vi "CupFinderV6.vi"() -> ()   [LabVIEW 2017]
panel:
  out "Y-Out":dbl
  out "X-Out":dbl
  out "CupPosition":T1(plugin-control)
  in  "File Path":path
  out "ImgToCrop":T1(plugin-control)
  out "Src Img":T1(plugin-control)
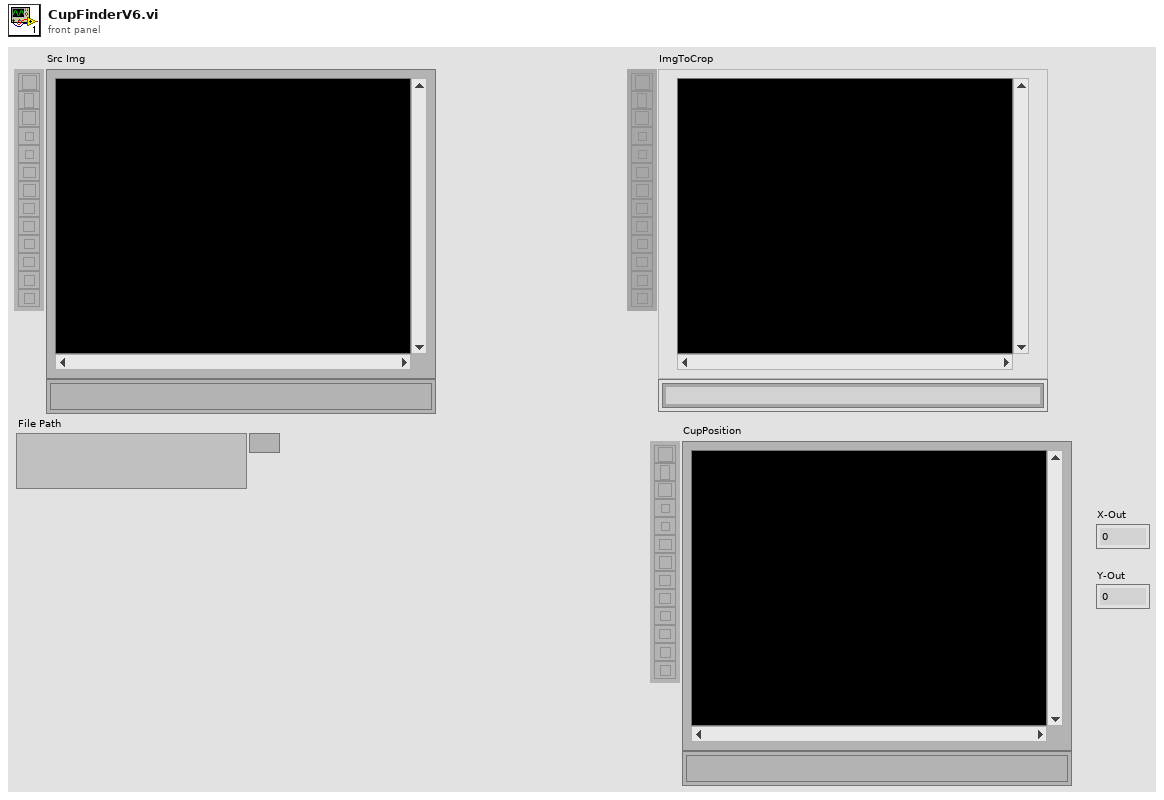
[diagram p1: front panel]
types:
  T1 = typedef "IMAQ Image.ctl" = refnum<image>
  T2 = typedef "Image Type" = u32
  T3 = cluster{"Position":cluster{"x":sgl, "y":sgl}, "Angle":sgl, "Scale":sgl, "Score":sgl, "Bounding Box":cluster{"x":sgl, "y":sgl}[]}[]
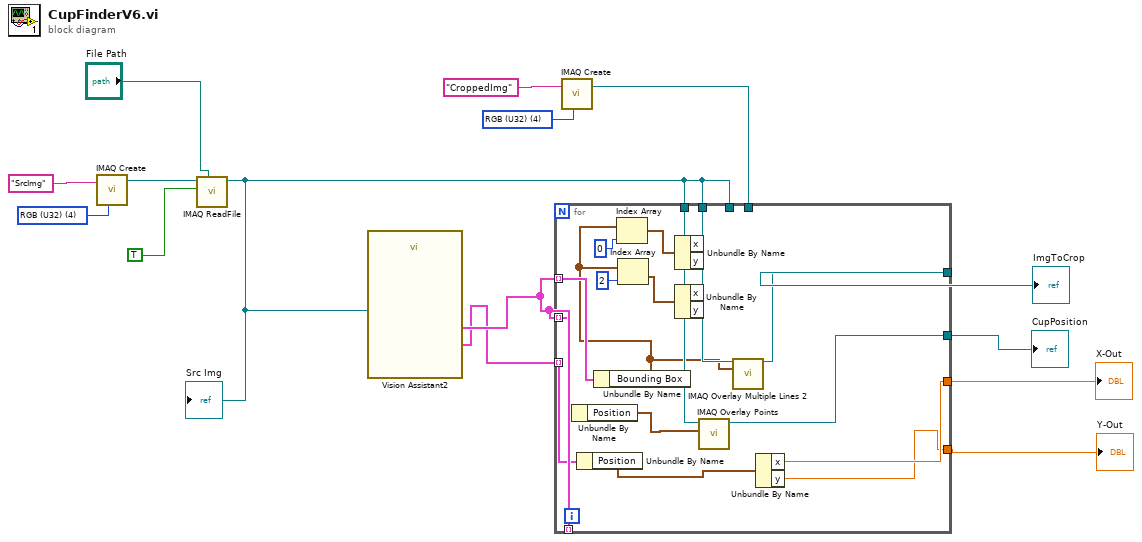
[diagram p0: block diagram]
diagram:
  w3 = T2 4 items=["Grayscale (U8)", "Grayscale (I16)", "Grayscale (SGL)", "Complex (CSG)", "RGB (U32)", "HSL (U32)", "RGB (U64)", "Grayscale (U16)"] ("Image Type")
  w14 = T2 4 items=["Grayscale (U8)", "Grayscale (I16)", "Grayscale (SGL)", "Complex (CSG)", "RGB (U32)", "HSL (U32)", "RGB (U64)", "Grayscale (U16)"] ("Image Type")
  n1 = call "IMAQ Create"("Image Name"="SrcImg", "Image Type"=w14) -> ("New Image"=w12:T1)  [unwired: 3 in, 1 out]
  n2 = call "IMAQ ReadFile"("File Path"="File Path", "Load Color Palette? (No)"=TRUE, "Image"=w12) -> ("Image Out"=w1:T1)  [unwired: 4 in, 4 out]
  "Src Img" <- w1
  n3 = call "Vision Assistant2"("Image In"=w1) -> ("Calibrated Matches (Pattern Matching 5)"=w5:T3, "Matches (Pattern Matching 5)"=w6:T3)  [unwired: 23 in, 2 out]
  n4 = call "IMAQ Create"("Image Name"="CroppedImg", "Image Type"=w3) -> ("New Image"=w2:T1)  [unwired: 3 in, 1 out]
  n5 = for {
    tunnel: [w22] -> w10
    tunnel: [w31] -> w9
    tunnel: [w29] -> w8
    tunnel: [w28] -> w7
    tunnel: w6 -> [_] mode=indexing
    tunnel: w1 -> [w27]
    tunnel: w1 -> [w26]
    tunnel: w6 -> [w24] mode=indexing
    tunnel: w6 -> [w21] mode=indexing
    tunnel: w5 -> [w23] mode=indexing
    tunnel: w2 -> [_]
    tunnel: w1 -> [_]
    n6 = Unbundle By Name(w24) -> ("Position"=w25:cluster{"x":sgl, "y":sgl})
    n7 = Unbundle By Name(w23) -> ("Position"=w30:cluster{"x":sgl, "y":sgl})
    n8 = Unbundle By Name(w21) -> ("Bounding Box"=w18:cluster{"x":sgl, "y":sgl}[])
    n9 = Index Array(array=w18, index=0) -> (element=w19:cluster{"x":sgl, "y":sgl})
    n10 = Index Array(array=w18, index=2) -> (element=w16:cluster{"x":sgl, "y":sgl})
    n11 = Unbundle By Name(w19) -> ()  [unwired: 2 out]
    n12 = Unbundle By Name(w16) -> ()  [unwired: 2 out]
    n13 = call "IMAQ Overlay Points"("Point"=w25, "Image"=w26) -> ("Image Out"=w31:T1)  [unwired: 8 in, 1 out]
    n14 = call "IMAQ Overlay Multiple Lines 2"("Image"=w27, "Line End Points"=w18) -> ("Image Out"=w22:T1)  [unwired: 12 in, 1 out]
    n15 = Unbundle By Name(w30) -> ("x"=w29:sgl, "y"=w28:sgl)
  }
  "ImgToCrop" <- w10
  "CupPosition" <- w9
  "X-Out" <- w8
  "Y-Out" <- w7
